vi "test pass 3.vi"(8 "error in (no error)":errorcluster, 11 "Passing test in":refnum<class "LUnit Test 11.lvclass">) -> (0 "error out":errorcluster, 3 "Passing test out":refnum<class "LUnit Test 11.lvclass">)   [LabVIEW 2020, in "LUnit Test 11.lvclass"]
uses:
  LUnit Test 11.lvclass
  C:/Program Files (x86)/National Instruments/LabVIEW 2020/vi.lib/Astemes/LUnit/Test Case.lvclass
  <vilib>/Astemes/LUnit/Test Case.lvclass/Test Case.ctl
  <vilib>/Astemes/LUnit/LUnit Assertion Result.lvclass/LUnit Assertion Result.ctl
  <vilib>/Astemes/LUnit/LUnit Test Case Result.lvclass/LUnit Test Case Result.ctl
  <vilib>/Astemes/LUnit/LUnit Method Result.lvclass/LUnit Method Result.ctl
  <vilib>/Astemes/LUnit/Palette/Fail.vi
  <vilib>/Astemes/LUnit/Palette/Pass.vi
  <vilib>/Astemes/LUnit/Set Assertion Type.vi
  <vilib>/Astemes/LUnit/Add test result.vi
  <vilib>/Astemes/LUnit/LUnit Write Passed.vi
  <vilib>/Astemes/LUnit/LUnit Write Message.vi
  <vilib>/Astemes/LUnit/LUnit Write Description.vi
  <vilib>/Astemes/LUnit/LUnit Write Assertion Type.vi
  <vilib>/Astemes/LUnit/LUnit Record Assertion Result.vi
  <vilib>/Astemes/LUnit/LUnit Aggregate Assertion Results.vi
  <vilib>/Astemes/LUnit/Assertion Result/LUnit Read Status.vi
  <vilib>/Astemes/LUnit/LUnit Read Message.vi
  <vilib>/Astemes/LUnit/LUnit Read Description.vi
  <vilib>/Astemes/LUnit/Method Result/LUnit Merge Status.vi
  <vilib>/Astemes/LUnit/LUnit Concatenate result strings.vi
  <vilib>/Astemes/LUnit/LUnit Assertion Result.lvclass
  <vilib>/Astemes/LUnit/Test Case.lvclass
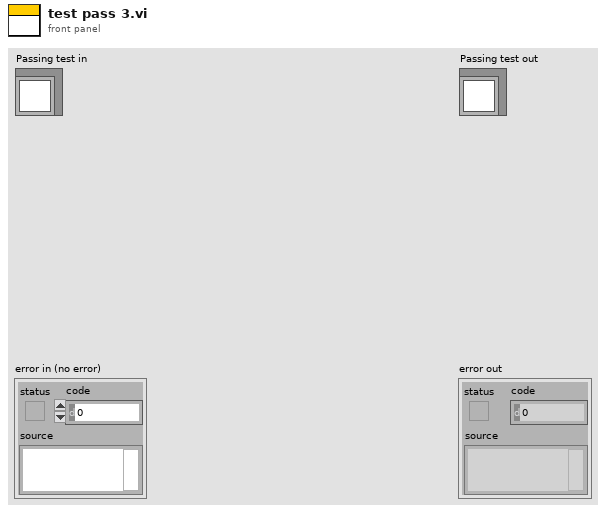
[diagram p1: front panel]
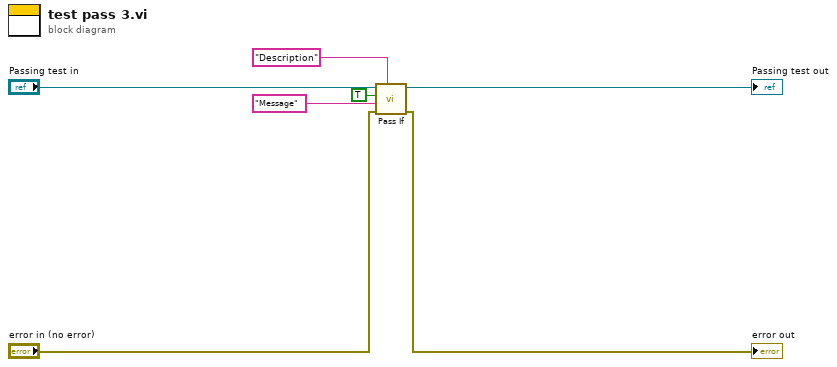
[diagram p0: block diagram]
diagram:
  n1 = call <vilib>:"Pass If.vi"("Description"="Description", "error in (no error)"="error in (no error)", "Message"="Message", "Pass?"=TRUE, "LUnit Test Case In"="Passing test in") -> ("error out"=→"error out":errorcluster, "LUnit Test Case Out"=→"Passing test out":refnum<class "LUnit Test 11.lvclass">)  [unwired: 5 in]
